vi "Write Force Measured.vi"(10 "Force Demand":T1 min=-888.0 max=888.0 format="%.2f", 11 "SystemController in":refnum<class "SystemController.lvclass">) -> (3 "SystemController out":refnum<class "SystemController.lvclass">)   [LabVIEW 2015]
uses:
  SystemController.lvclass
  Typedefs/ForceDemand.ctl
  Typedefs/M1M3SSSTypedefs.lvlib
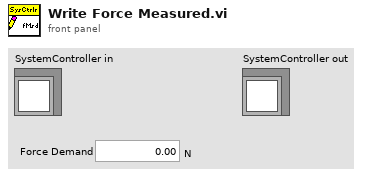
[diagram p1: front panel]
types:
  T1 = typedef "M1M3SSSTypedefs.lvlib/ForceDemand.ctl" = dbl[unit]
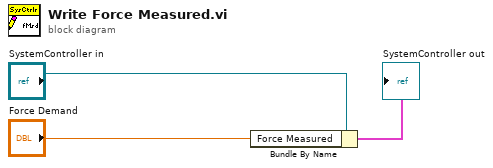
[diagram p0: block diagram]
diagram:
  n1 = Bundle By Name(cluster="SystemController in", "Force Measured"="Force Demand") -> (→"SystemController out":cluster{})
